vi "Fetch (Unscaled Waveform).vi"(7 "Segment Index (0)":i32 format="%.0g", 8 "error in (no error)":errorcluster, 9 "Maximum Time (10000ms)":u32, 10 "Channel (1: Channel 1)":u16(ring) items=["Channel 1", "Channel 2", "Channel 3", "Channel 4", "Function 1", "Function 2", "Function 3", "Function 4", "Memory 1", "Memory 2", "Memory 3", "Memory 4"], 11 "VISA resource name":refnum<visa-resource-name>) -> (0 "error out":errorcluster, 1 "dt":dbl, 2 "t0":dbl, 3 "VISA resource name out":refnum<visa-resource-name>, 4 "Waveform Data":i8[](array[numeric]))   [LabVIEW 2009, in "Agilent 8000 Series.lvlib"]
doc: "Returns the raw data that an oscilloscope acquires for a channel you specify. An acquisition that you initiate before calling this VI generates the waveform. If the sampling mode is set to segment, you can set the <B>Segment Index</B>.The waveform data you fetch from the oscilloscope is an interger value, expressed in waveform data point level. Data width is of one byte so the data range is 0 to 255.You choose to use this VI when you want a relative fast fetching speed as well as output data expressed in waveform data point level. If you want output waveform data expressed in unit of volts, you could use this VI and manually scale the output data, or you could choose to use the <B>Fetch (Waveform)</B> VI.\n\nYou first enable channels with the Configure Channel VI. Then you use the Initiate VI to start an acquisition on the enabled channels. An oscilloscope concurrently acquires waveforms for these channels. You must call the Fetch VI separately to obtain waveforms for each enabled channel.\nHowever, you also can call the Read VI instead of using the above low-level VIs.\n\n<B>Note</B>: Use the Fetch (Unscaled Waveform) VI only with other low-level VIs, such as the Initiate VI, the Abort VI, and the Fetch Measurement VI. High-level VIs, such as the Read VI, automatically incorporate the functions of the Initiate VI and the Fetch VI. The Fetch VI does not check the status of an instrument."
uses:
  Agilent 8000 Series.lvlib
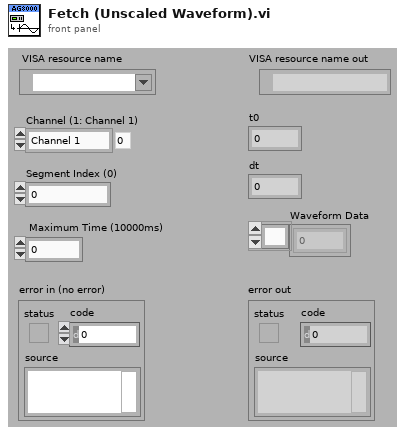
[diagram p1: front panel]
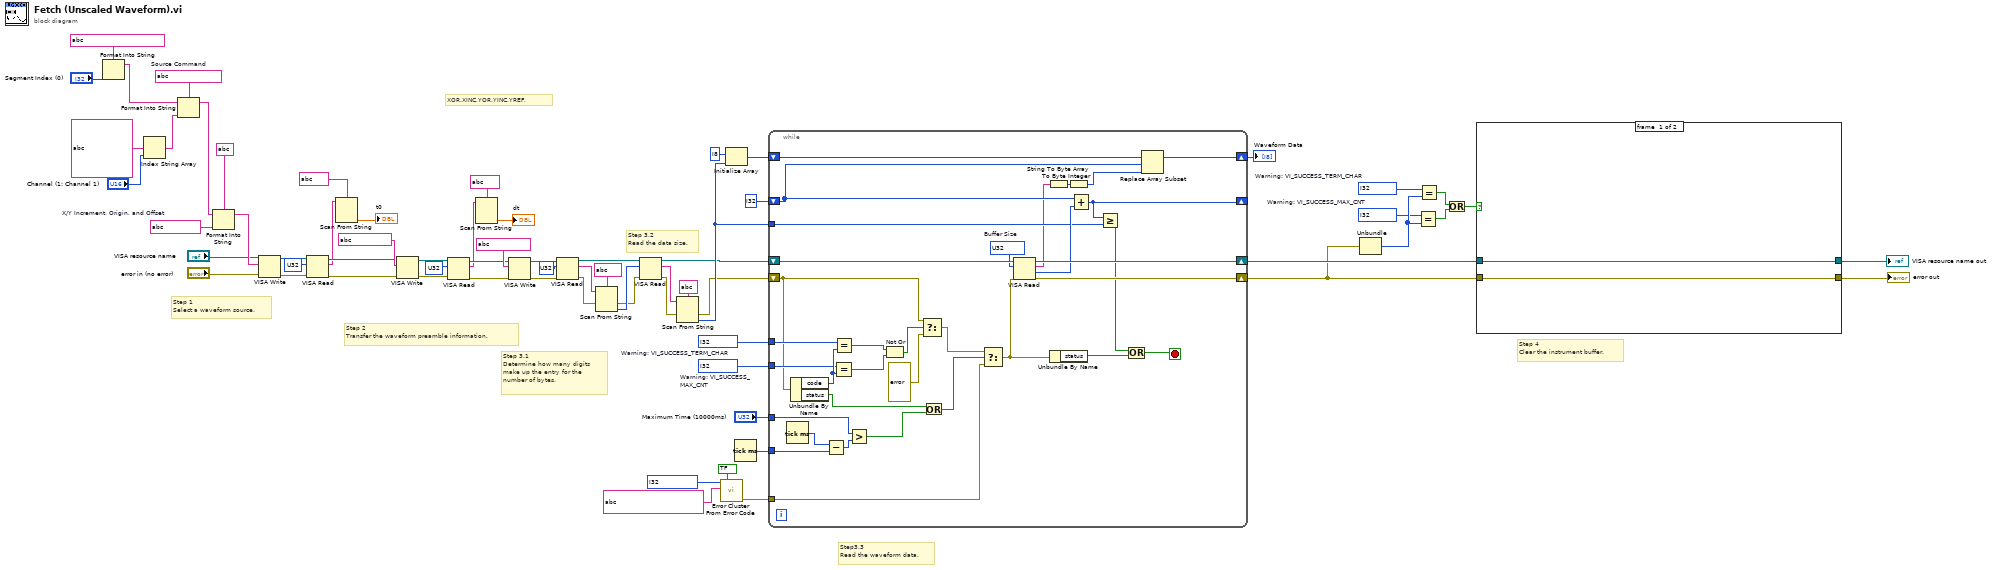
[diagram p0: block diagram]
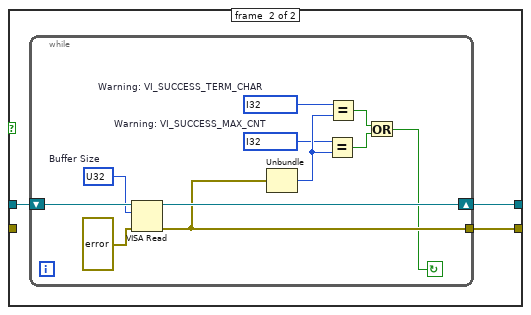
[diagram p2: hidden frame]
diagram:
  w45 = i32 ?  # Warning: VI_SUCCESS_MAX_CNT
  w44 = i32 ?  # Warning: VI_SUCCESS_TERM_CHAR
  w37 = i32 ?  # Warning: VI_SUCCESS_MAX_CNT
  w36 = i32 ?  # Warning: VI_SUCCESS_TERM_CHAR
  w65 = string ?  # Source Command
  w58 = string ?  # X/Y Increment, Origin, and Offset
  # "Step 4    \nClear the instrument buffer."
  # "Step3.3   \nRead the waveform data."
  # "Step 3.2     \nRead the data size."
  # "Step 3.1     \nDetermine how many digits\nmake up the entry for the \nnumber of bytes."
  # "Step 1       \nSelect a waveform source."
  # "Step 2\nTransfer the waveform preamble information."
  # "XOR,XINC,YOR,YINC,YREF,"
  n1 = Format Into String(format string=string ?, "Segment Index (0)") -> (resulting string=w53:string)  [unwired: 2 in, 1 out]
  n2 = Index String Array(1:"Channel (1: Channel 1)", 2:string[] ?) -> (0:w59:string)  [unwired: 1 in]
  n3 = Format Into String(format string=w65, initial string=w53, w59) -> (resulting string=w63:string)  [unwired: 1 in, 1 out]
  n4 = Format Into String(format string=string ?, initial string=w63, w58) -> (resulting string=w62:string)  [unwired: 1 in, 1 out]
  n5 = VISA Write(VISA resource name="VISA resource name", write buffer=w62, error in (no error)="error in (no error)") -> (VISA resource name out=w68:refnum<visa-resource-name>, error out=w67:errorcluster)  [unwired: 1 out]
  n6 = VISA Read(VISA resource name=w68, byte count=u32 ?, error in (no error)=w67) -> (VISA resource name out=w13:refnum<visa-resource-name>, read buffer=w6:string, error out=w12:errorcluster)  [unwired: 1 out]
  n7 = Scan From String(format string=string ?, input string=w6) -> (output 1=→"t0":dbl)  [unwired: 3 in, 3 out]
  n8 = VISA Write(VISA resource name=w13, write buffer=string ?, error in (no error)=w12) -> (VISA resource name out=w11:refnum<visa-resource-name>, error out=w10:errorcluster)  [unwired: 1 out]
  n9 = VISA Read(VISA resource name=w11, byte count=u32 ?, error in (no error)=w10) -> (VISA resource name out=w9:refnum<visa-resource-name>, read buffer=w4:string, error out=w8:errorcluster)  [unwired: 1 out]
  n10 = Scan From String(format string=string ?, input string=w4) -> (output 1=→"dt":dbl)  [unwired: 3 in, 3 out]
  n11 = VISA Write(VISA resource name=w9, write buffer=string ?, error in (no error)=w8) -> (VISA resource name out=w20:refnum<visa-resource-name>, error out=w19:errorcluster)  [unwired: 1 out]
  n12 = VISA Read(VISA resource name=w20, byte count=u32 ?, error in (no error)=w19) -> (VISA resource name out=w26:refnum<visa-resource-name>, read buffer=w23:string, error out=w22:errorcluster)  [unwired: 1 out]
  n13 = Scan From String(format string=string ?, input string=w23, error in=w22) -> (error out=w25:errorcluster, output 1=w52:i32)  [unwired: 2 in, 2 out]
  n14 = VISA Read(VISA resource name=w26, byte count=w52, error in (no error)=w25) -> (VISA resource name out=w30:refnum<visa-resource-name>, read buffer=w29:string, error out=w27:errorcluster)  [unwired: 1 out]
  n15 = Scan From String(format string=string ?, input string=w29, error in=w27) -> (error out=w31:errorcluster, output 1=w35:i32)  [unwired: 2 in, 2 out]
  n16 = call <vilib>:"Error Cluster From Error Code.vi"("show call chain? (False)"=bool ?, "error message (\"\")"=string ? ("error message (\"\")"), "error code (0)"=i32 ?) -> ("error out"=w43:errorcluster)  [unwired: 6 in]
  n17 = Initialize Array(i8 ? ("element"), w35) -> (w33:i8[])
  n18 = Tick Count (ms)() -> (millisecond timer value=w42:u32)
  n19 = while {
    shift-right: [w97] -> w50
    shift-left: w31 -> [w84]
    shift-right: [w102] -> w51
    shift-left: w30 -> [w101]
    shift-right: [w98] -> w15
    shift-left: w33 -> [w99]
    shift-right: [w94] -> _
    shift-left: i32 ? ("index") -> [w95]
    tunnel: w35 -> [w93]
    tunnel: w36 -> [w86]
    tunnel: w37 -> [w85]
    tunnel: "Maximum Time (10000ms)" -> [w81]
    tunnel: w42 -> [w80]
    tunnel: w43 -> [w75]
    stop <- w72 stop-if-true
    w100 = u32 ?  # Buffer Size
    n20 = Tick Count (ms)() -> (millisecond timer value=w82:u32)
    n21 = Unbundle By Name(w84) -> ("code"=w87:i32, "status"=w79:bool)
    n22 = Subtract(x=w82, y=w80) -> (x-y=w83:u32)
    n23 = Equal?(x=w85, y=w87) -> (x = y?=w90:bool)
    n24 = Equal?(x=w86, y=w87) -> (x = y?=w91:bool)
    n25 = Greater?(x=w81, y=w83) -> (0:w78:bool)
    n26 = Not Or(1:w90, 2:w91) -> (0:w89:bool)
    n27 = Select(t=w84, s=w89, f=errorcluster ? ("error in (no error)")) -> (s? t:f=w77:errorcluster)
    n28 = Or(x=w79, y=w78) -> (x .or. y?=w76:bool)
    n29 = Select(t=w77, s=w76, f=w75) -> (s? t:f=w74:errorcluster)
    n30 = VISA Read(VISA resource name=w101, byte count=w100, error in (no error)=w74) -> (VISA resource name out=w102:refnum<visa-resource-name>, read buffer=w71:string, return count=w96:u32, error out=w97:errorcluster)
    n31 = String To Byte Array(string=w71) -> (unsigned byte array=w70:u8[])
    n32 = Unbundle By Name(w74) -> ("status"=w73:bool)
    n33 = To Byte Integer(number=w70) -> (8bit integer=w69:i8[])
    n34 = Add(x=w95, y=w96) -> (x+y=w94:u32)
    n35 = Greater Or Equal?(x=w94, y=w93) -> (x >= y?=w92:bool)
    n36 = Compound Arithmetic op=OR(w92, w73) -> (w72:bool)
    n37 = Replace Array Subset(array=w99, new element=w69, index=w95) -> (w98:i8[])
  }
  "Waveform Data" <- w15
  n38 = Unbundle(w50) -> ("code"=w46:i32)  [unwired: 2 out]
  n39 = Equal?(x=w45, y=w46) -> (x = y?=w48:bool)
  n40 = Equal?(x=w44, y=w46) -> (x = y?=w49:bool)
  n41 = Or(x=w49, y=w48) -> (x .or. y?=w47:bool)
  n42 = case shown="True" w47 {
    tunnel: w51 -> [w104 w107]
    tunnel: w50 -> [w103 _]
    tunnel: [w104 w106] -> w17
    tunnel: [w103 w105] -> w16
    frame #0 {
    }
    frame #1 {
      n43 = while {
        shift-right: [w117] -> w106
        shift-left: w107 -> [w118]
        tunnel: [w110] -> w105
        stop <- w109 continue-if-true
        w112 = i32 ?  # Warning: VI_SUCCESS_MAX_CNT
        w111 = i32 ?  # Warning: VI_SUCCESS_TERM_CHAR
        w116 = u32 ?  # Buffer Size
        n44 = VISA Read(VISA resource name=w118, byte count=w116, error in (no error)=errorcluster ?) -> (VISA resource name out=w117:refnum<visa-resource-name>, error out=w110:errorcluster)  [unwired: 2 out]
        n45 = Unbundle(w110) -> ("code"=w113:i32)  [unwired: 2 out]
        n46 = Equal?(x=w112, y=w113) -> (x = y?=w114:bool)
        n47 = Equal?(x=w111, y=w113) -> (x = y?=w115:bool)
        n48 = Or(x=w115, y=w114) -> (x .or. y?=w109:bool)
      }
    }
  }
  "error out" <- w16
  "VISA resource name out" <- w17
